vi "SetMenu.vi"(8 "error in (no error)":errorcluster caption="错误输入（无错误）", 10 "菜单引用":refnum<k9>, 11 "TrendPlot 输入":refnum<class "TrendPlot.lvclass">) -> (0 "error out":errorcluster caption="错误输出", 3 "TrendPlot 输出":refnum<class "TrendPlot.lvclass">)   [LabVIEW 2018, in "DataDisplay.lvlib" / "TrendPlot.lvclass"]
uses:
  TrendPlot.lvclass
  TrendPlot.lvclass/TrendPlot.ctl
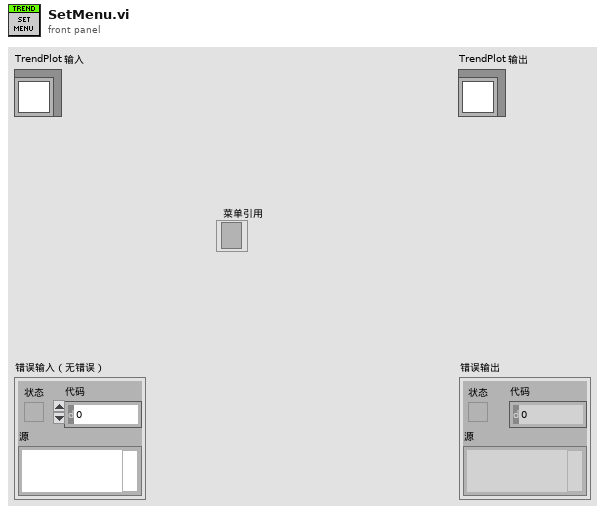
[diagram p1: front panel]
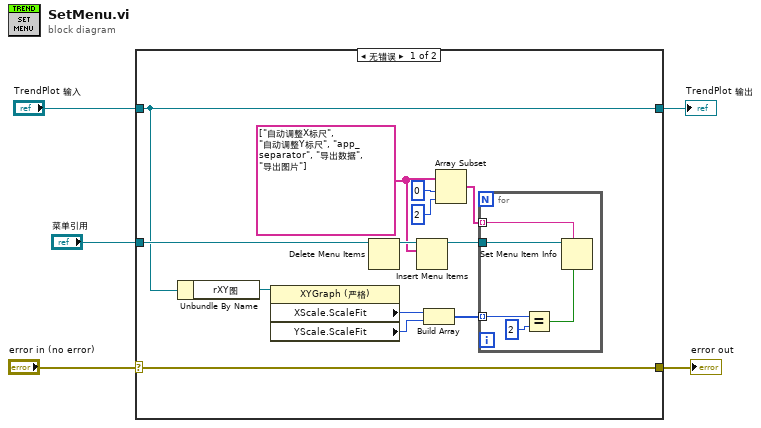
[diagram p0: block diagram]
diagram:
  n1 = case shown="无错误" "error in (no error)" {
    selector: "error in (no error)" -> [w18 w25]
    tunnel: [w18 w25] -> w4
    tunnel: [w14 w24] -> w2
    tunnel: "TrendPlot 输入" -> [w14 w24]
    tunnel: "菜单引用" -> [w16 _]
    frame No Error {
      w15 = string[] ["自动调整X标尺", "自动调整Y标尺", "app_separator", "导出数据", "导出图片"] ("项标识符")
      n2 = Unbundle By Name(w14) -> ("rXY图"=w13:refnum<vi>)
      n3 = property class="XYGraph (严格)"(reference=w13) -> ("XScale.ScaleFit"=w12:u8, "YScale.ScaleFit"=w11:u8)  [unwired: 1 in, 2 out]
      n4 = Delete Menu Items(9:w16) -> (3:w17:refnum<k9>)  [unwired: 3 in, 1 out]
      n5 = Insert Menu Items(8:w15, 9:w17) -> (3:w6:refnum<k9>)  [unwired: 4 in, 2 out]
      n6 = Build Array(w12, w11) -> (w9:u8[])
      n7 = Array Subset(array=w15, index=0 ("索引"), length=2 ("长度")) -> (w10:string[])
      n8 = for {
        tunnel: w10 -> [w23] mode=indexing
        tunnel: w9 -> [w22] mode=indexing
        tunnel: w6 -> [w19]
        n9 = Equal?(x=w22, y=u8 2) -> (x = y?=w20:bool)
        n10 = Set Menu Item Info(6:w20, 7:w23, 11:w19) -> ()  [unwired: 4 in, 2 out]
      }
    }
    frame Error {
    }
  }
  "error out" <- w4
  "TrendPlot 输出" <- w2
